vi "valve_control_output.vi"(0 "STOP! Refnum":refnum<vi>, 2 "Voltage Arr Refnum":refnum<vi>, 4 "Liquid channel":tag="cDAQ1Mod4/ao3", 5 "Vapor channel":tag="cDAQ1Mod4/ao2") -> ()   [LabVIEW 2017]
uses:
  <resource>/objmgr/daqmx.rc
  <vilib>/DAQmx/write.llb/DAQmx Write (Analog 1D DBL NChan 1Samp).vi
  <vilib>/DAQmx/create/channels.llb/DAQmx Create Channel (AO-Voltage-Basic).vi
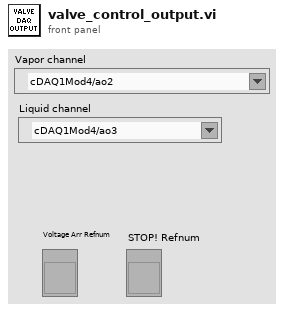
[diagram p1: front panel]
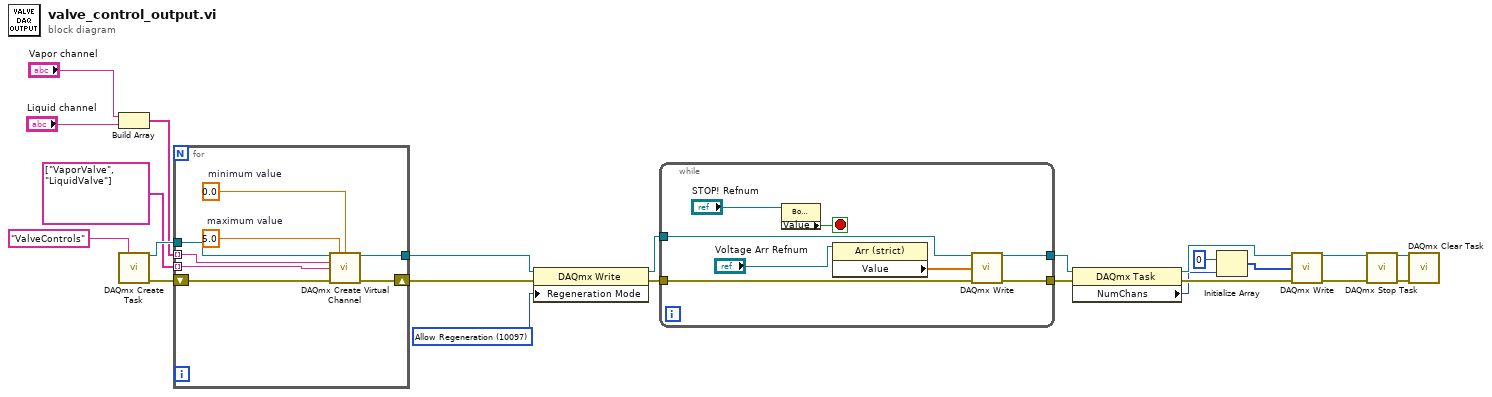
[diagram p0: block diagram]
diagram:
  w17 = 10097 items=["Allow Regeneration"=10097, "Do Not Allow Regeneration"=10158] ("RegenMode")
  n1 = Build Array("Vapor channel", "Liquid channel") -> (w18:tag[])
  n2 = call <vilib>:"DAQmx Create Task.vi"("new task name"="ValveControls") -> ("task out"=w23:refnum<k21>, "error out"=w22:errorcluster)  [unwired: 13 in]
  n3 = for {
    tunnel: w23 -> [w31]
    shift-right: [w24] -> w13
    shift-left: w22 -> [w30]
    tunnel: string[] ["VaporValve", "LiquidValve"] -> [w29] mode=indexing
    tunnel: w18 -> [w28] mode=indexing
    tunnel: [w25] -> w14
    w26 = 0.0  # minimum value
    w27 = 5.0  # maximum value
    n4 = call-poly <vilib>:"DAQmx Create Virtual Channel.vi"("task in"=w31, "maximum value"=w27, "minimum value"=w26, "physical channels"=w28, "name to assign"=w29, "error in"=w30) -> ("task out"=w25:refnum<k21>, "error out"=w24:errorcluster)  [unwired: 8 in]
  }
  n5 = property class="DAQmx Write"(reference=w14, error in=w13, "Regeneration Mode"=w17) -> (reference out=w11:refnum<k21>, error out=w12:errorcluster)
  n6 = while {
    tunnel: w11 -> [w34]
    tunnel: [w33] -> w4
    tunnel: w12 -> [w37]
    tunnel: [w32] -> w7
    stop <- w38 stop-if-true
    n7 = property class="Bool (strict)"(reference="STOP! Refnum") -> ("Value"=w38:bool)  [unwired: 1 in, 2 out]
    n8 = property class="Arr (strict)"(reference="Voltage Arr Refnum") -> ("Value"=w35:dbl[])  [unwired: 1 in, 2 out]
    n9 = call-poly <vilib>:"DAQmx Write.vi"("task/channels in"=w34, "data"=w35, "error in"=w37) -> ("task out"=w33:refnum<k21>, "error out"=w32:errorcluster)  [unwired: 10 in, 1 out]
  }
  n10 = property class="DAQmx Task"(reference=w4, error in=w7) -> (reference out=w3:refnum<k21>, error out=w2:errorcluster, "NumChans"=w1:u32)
  n11 = Initialize Array(u32 0 ("element"), w1) -> (w5:u32[])
  n12 = call-poly <vilib>:"DAQmx Write.vi"("task/channels in"=w3, "data"=w5, "error in"=w2) -> ("task out"=w9:refnum<k21>, "error out"=w8:errorcluster)  [unwired: 10 in, 1 out]
  n13 = call <vilib>:"DAQmx Stop Task.vi"("task/channels in"=w9, "error in"=w8) -> ("task out"=w16:refnum<k21>, "error out"=w15:errorcluster)  [unwired: 12 in]
  n14 = call <vilib>:"DAQmx Clear Task.vi"("task in"=w16, "error in"=w15) -> ()  [unwired: 13 in, 1 out]
